vi "Assembler.vi"() -> ()   [LabVIEW 2017, in "User Manager Application.lvlib"]
uses:
  User Manager Application.lvlib
  <vilib>/ActorFramework/Message Enqueuer/Message Priority.ctl
  <vilib>/gpm_packages/@cs/mva-viewable/Source/IViewable/IViewable/View Position Enum.ctl
  ViewModel/ViewModel/ViewModel.lvclass
  C:/Program Files/National Instruments/LabVIEW 2017/vi.lib/gpm_packages/@cs/mva-core/Source/IObserver/IObserver/IObserver.lvclass
  C:/Program Files/National Instruments/LabVIEW 2017/vi.lib/gpm_packages/@cs/mva-viewable/Source/IViewModel/IViewModel/IViewModel.lvclass
  C:/Program Files/National Instruments/LabVIEW 2017/vi.lib/ActorFramework/Actor/Actor.lvclass
  View Manager/View Manager/View Manager.lvclass
  C:/Program Files/National Instruments/LabVIEW 2017/vi.lib/gpm_packages/@cs/mva-viewable/Source/IViewManager/IViewManager/IViewManager.lvclass
  C:/Program Files/National Instruments/LabVIEW 2017/vi.lib/gpm_packages/@cs/mva-viewable/Source/IViewable/IViewable/IViewable.lvclass
  User Manager Model/User Manager Model/User Manager Model.lvclass
  C:/Program Files/National Instruments/LabVIEW 2017/vi.lib/gpm_packages/@cs/mva-core/Source/IModel/IModel/IModel.lvclass
  Login View/Login View/Login View.lvclass
  User Manager View/User Manager View/User Manager View.lvclass
  <vilib>/gpm_packages/@cs/mva-core/Source/Mediator/Mediator/Mediator.lvclass
  C:/Program Files/National Instruments/LabVIEW 2017/vi.lib/gpm_packages/@cs/mva-core/Source/IMediator/IMediator/IMediator.lvclass
  <vilib>/gpm_packages/@cs/mva-core/Source/IModel/IModel/IModel.lvclass
  <vilib>/gpm_packages/@cs/mva-viewable/Source/IViewManager/IViewManager Messages/Launch Nested Views Msg/Launch Nested Views Msg.lvclass/Launch Nested Views Msg.ctl
  <vilib>/gpm_packages/@cs/mva-viewable/Source/IViewManager/IViewManager/IViewManager.lvclass/IViewManager.ctl
  <vilib>/gpm_packages/@cs/event-logger/Source/Composed Log/LoggerReference/LoggerReference.lvclass/LoggerReference.ctl
  <vilib>/gpm_packages/@cs/mva-core/Source/IObserver/IObserver/IObserver.lvclass/IObserver.ctl
  <vilib>/gpm_packages/@cs/mva-core/Source/IMediator/IMediator/IMediator.lvclass/IMediator.ctl
  <vilib>/gpm_packages/@cs/mva-viewable/Source/IViewModel/IViewModel/IViewModel.lvclass/IViewModel.ctl
  <vilib>/gpm_packages/@cs/mva-viewable/Source/IViewable/IViewable Messages/Open Front Panel Msg/Open Front Panel Msg.lvclass/Open Front Panel Msg.ctl
  <vilib>/ActorFramework/Message Enqueuer/Message Enqueuer.lvclass/Message Enqueuer.ctl
  14d4f322-1a71-411e-b970-6e06ce8b6413.vi
  <vilib>/gpm_packages/@cs/mva-viewable/Source/IViewManager/IViewManager Messages/Launch Nested Views Msg/Pack Launch Nested Views Msg.vi
  14d4f322-1a71-411e-b970-6e06ce8b6413.vi/08d843f9-281e-434a-81fc-1a5d90edc2f4.vi
  <vilib>/gpm_packages/@cs/mva-core/Source/IObserver/IObserver/Configure Observer Logging.vi
  <vilib>/gpm_packages/@cs/mva-viewable/Source/IViewModel/IViewModel/Write Startup Model-View Configuration.vi
  <vilib>/gpm_packages/@cs/mva-core/Source/IMediator/IMediator/Configure Mediator.vi
  <vilib>/ActorFramework/Message Enqueuer/Enqueue.vi
  <vilib>/gpm_packages/@cs/event-logger/Source/Composed Log/LoggerReference/Return Aggregate Queues.vi
  <vilib>/gpm_packages/@cs/event-logger/Source/Composed Log/LoggerReference/Add Aggregate Log.vi
  14d4f322-1a71-411e-b970-6e06ce8b6413.vi/08d843f9-281e-434a-81fc-1a5d90edc2f4.vi/e0167d68-300f-4ef6-b43f-639807bb0888.vi
  <vilib>/gpm_packages/@cs/mva-viewable/Source/IViewManager/IViewManager/Write Startup Launch Nested Views Msg.vi
  <vilib>/gpm_packages/@cs/event-logger/Source/Composed Log/LoggerReference/Send Add Sink.vi
  <vilib>/gpm_packages/@cs/event-logger/Source/Text File Sink/Text File Sink.lvclass
  C:/Program Files/National Instruments/LabVIEW 2017/vi.lib/gpm_packages/@cs/event-logger/Source/Composed Log/Log Sink/Log Sink.lvclass
  <vilib>/gpm_packages/@cs/mva-viewable/Source/IViewModel/IViewModel/IViewModel.lvclass
  <vilib>/gpm_packages/@cs/mva-viewable/Source/IViewable/IViewable Messages/Open Front Panel Msg/Open Front Panel Msg.lvclass
  C:/Program Files/National Instruments/LabVIEW 2017/vi.lib/ActorFramework/Message/Message.lvclass
  <vilib>/gpm_packages/@cs/event-logger/Source/Composed Log/Application Logger/Launch Worker Loop.vi
  <vilib>/gpm_packages/@cs/event-logger/Source/Composed Log/LoggerReference/Initialize Logger Instance.vi
  <vilib>/ActorFramework/Message Priority Queue/Priority Enqueue.vi
  <vilib>/gpm_packages/@cs/mva-viewable/Source/IViewManager/IViewManager Messages/Launch Nested Views Msg/Launch Nested Views Msg.lvclass
  <vilib>/gpm_packages/@cs/event-logger/Source/Composed Log/LoggerReference/LoggerReference.lvclass
  <vilib>/gpm_packages/@cs/event-logger/Source/Composed Log/IErrorFormat/IErrorFormat.lvclass
  <vilib>/gpm_packages/@cs/event-logger/Source/Composed Log/Log Sink/Log Sink.lvclass
  <vilib>/gpm_packages/@cs/mva-viewable/Source/IViewable/IApplicationStyle/IApplicationStyle.lvclass
  <vilib>/ActorFramework/Actor/Actor.lvclass
  <vilib>/ActorFramework/Message Enqueuer/Message Enqueuer.lvclass
  <vilib>/gpm_packages/@cs/mva-viewable/Source/IViewable/IViewable/IViewable.lvclass
  <vilib>/gpm_packages/@cs/mva-viewable/Source/IViewManager/IViewManager/IViewManager.lvclass
panel:
  out "error out":errorcluster
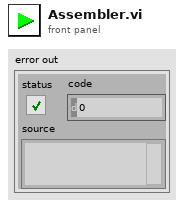
[diagram p1: front panel]
types:
  T1 = typedef "IViewable.lvlib/IViewable.lvclass/View Position Enum.ctl" = enum16{"Centered", "Maximized", "Minimized", "Custom", "Unchanged"}
  T2 = typedef "Actor Framework.lvlib/Message Enqueuer.lvclass/Message Priority.ctl" = enum16{"Low", "Normal", "High"}
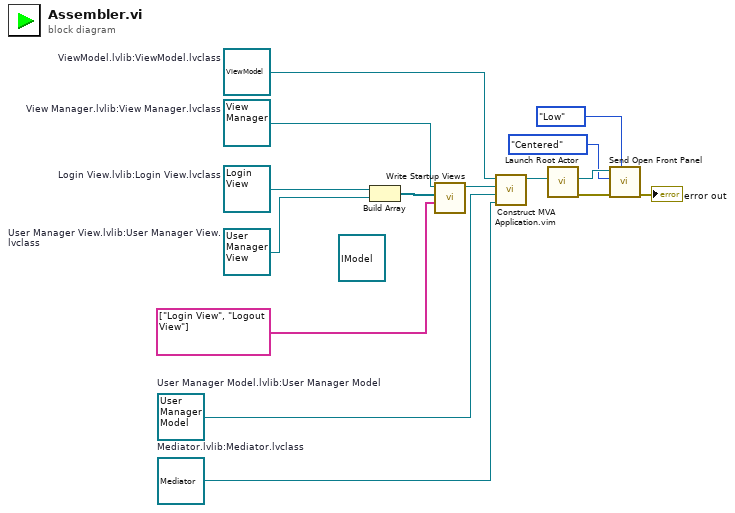
[diagram p0: block diagram]
diagram:
  (unwired) refnum<class "IModel.lvclass"> refnum ("Model Type")
  w2 = refnum<class "Mediator.lvclass"> refnum  # Mediator.lvlib:Mediator.lvclass
  w5 = refnum<class "User Manager View.lvclass"> refnum  # User Manager View.lvlib:User Manager View.lvclass
  w6 = refnum<class "Login View.lvclass"> refnum  # Login View.lvlib:Login View.lvclass
  w1 = refnum<class "User Manager Model.lvclass"> refnum  # User Manager Model.lvlib:User Manager Model
  w7 = refnum<class "View Manager.lvclass"> refnum  # View Manager.lvlib:View Manager.lvclass
  w9 = refnum<class "ViewModel.lvclass"> refnum  # ViewModel.lvlib:ViewModel.lvclass
  n1 = Build Array(w6, w5) -> (w4:refnum<class "IViewable.lvclass">[])
  n2 = call <vilib>:"Write Startup Views.vi"("View Labels"=string[] ["Login View", "Logout View"], "Startup Views"=w4, "IViewManager in"=w7) -> ("IViewManager out"=w8:refnum<class "View Manager.lvclass">)  [unwired: 8 in]
  n3 = call "Construct MVA Application.vim"("Mediator Type"=w2, "Model Type"=w1, "Startup View Configuration"=w8, "IViewModel In"=w9) -> ("IViewModel Out"=w10:refnum<class "ViewModel.lvclass">)  [unwired: 7 in]
  n4 = call <vilib>:"Launch Root Actor.vi"("Actor"=w10) -> ("error out"=w11:errorcluster, "Actor's Enqueuer"=w15:refnum<class "Message Enqueuer.lvclass">)  [unwired: 9 in]
  n5 = call <vilib>:"Send Open Front Panel.vi"("Message Priority (Normal)"=Message_Priority."Low", "error in (no error)"=w11, "Position"=View_Position_Enum."Centered", "Message Enqueuer"=w15) -> ("error out"=→"error out":errorcluster)  [unwired: 6 in, 1 out]
